vi "Write Menu Value.vi"(8 "Error In":errorcluster, 9 "Menu Write choice":T1) -> (0 "Error Out":errorcluster, 1 "Right Menu":T2, 2 "Left Menu":T2)   [LabVIEW 2019]
doc: "This VI is used to write values to menu."
uses:
  Controls/Write Menu.ctl
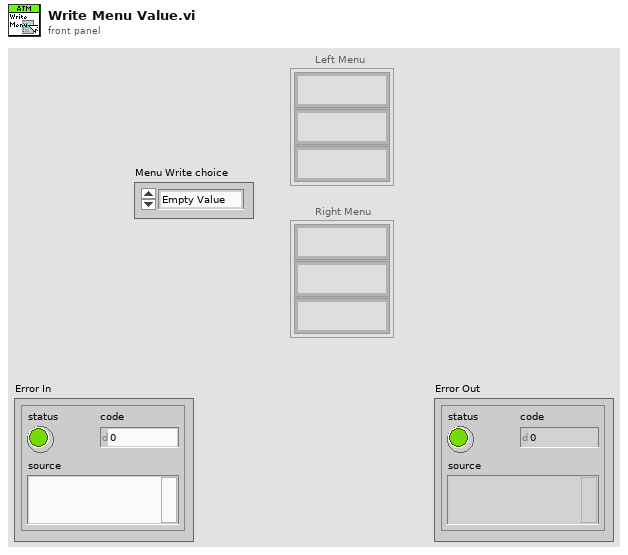
[diagram p1: front panel]
types:
  T1 = typedef "Write Menu.ctl" = enum16{"Empty Value", "Standard Value"}
  T2 = cluster{"RFS String":string, "RFS String 2":string, "RFS String 3":string}
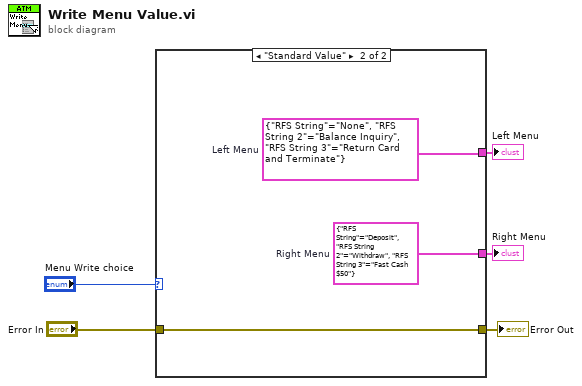
[diagram p0: block diagram]
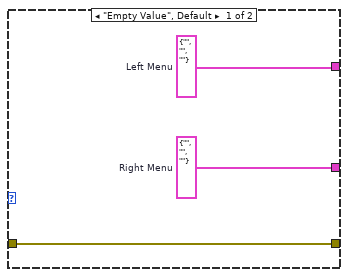
[diagram p2: hidden frame]
diagram:
  n1 = case shown="\"Standard Value\"" "Menu Write choice" {
    tunnel: [w8 w11] -> w3
    tunnel: [w7 w10] -> w4
    tunnel: "Error In" -> [w6 w9]
    tunnel: [w6 w9] -> w1
    frame "Empty Value", Default {
      w8 = T2 {"RFS String"="", "RFS String 2"="", "RFS String 3"=""}  # Left Menu
      w7 = T2 {"RFS String"="", "RFS String 2"="", "RFS String 3"=""}  # Right Menu
    }
    frame "Standard Value" {
      w11 = T2 {"RFS String"="None", "RFS String 2"="Balance Inquiry", "RFS String 3"="Return Card and Terminate"}  # Left Menu
      w10 = T2 {"RFS String"="Deposit", "RFS String 2"="Withdraw", "RFS String 3"="Fast Cash $50"}  # Right Menu
    }
  }
  "Left Menu" <- w3
  "Right Menu" <- w4
  "Error Out" <- w1
